vi "Body_LS(SubVI).vi"(3 "error in":errorcluster caption="error in\nerror in", 4 "문자열":string, 5 "VISA resource name out 2":refnum<visa-resource-name>) -> (0 "error out":errorcluster, 1 "read buffer":string, 2 "VISA resource name out":refnum<visa-resource-name>)   [LabVIEW 2014]
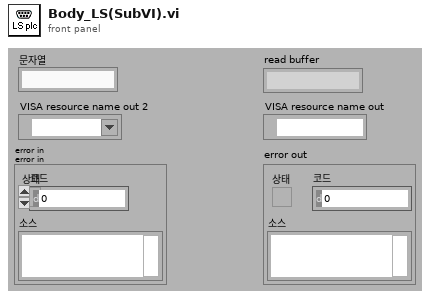
[diagram p1: front panel]
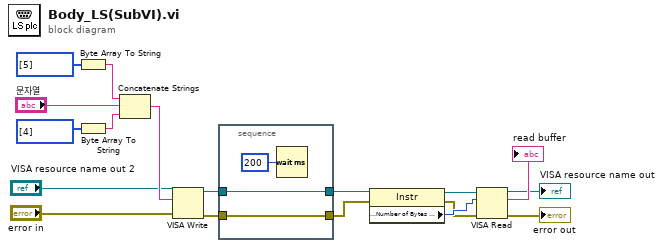
[diagram p0: block diagram]
diagram:
  n1 = Byte Array To String(unsigned byte array=u8[] [5] ("부호없는 바이트 배열")) -> (string=w14:string)
  n2 = Byte Array To String(unsigned byte array=u8[] [4] ("부호없는 바이트 배열")) -> (string=w13:string)
  n3 = Concatenate Strings(w14, "문자열", w13) -> (w18:string)
  n4 = VISA Write(VISA resource name="VISA resource name out 2", write buffer=w18, error in (no error)="error in") -> (VISA resource name out=w3:refnum<visa-resource-name>, error out=w4:errorcluster)  [unwired: 1 out]
  n5 = stacked-sequence {
    tunnel: w3 -> [w21]
    tunnel: w4 -> [w20]
    tunnel: [w21] -> w5
    tunnel: [w20] -> w6
    frame #0 {
      n6 = Wait (ms)(milliseconds to wait=u32 200 ("기다릴 ms")) -> ()  [unwired: 1 out]
    }
  }
  n7 = property class="Instr"(reference=w5, error in=w6) -> (reference out=w7:refnum<visa-resource-name>, error out=w8:errorcluster, "Serial Settings:Number of Bytes at Serial Port"=w11:u32)
  n8 = VISA Read(VISA resource name=w7, byte count=w11, error in (no error)=w8) -> (VISA resource name out=→"VISA resource name out":refnum<visa-resource-name>, read buffer=→"read buffer":string, error out=→"error out":errorcluster)  [unwired: 1 out]
